vi "FPGA_DIOWritePWMMinHigh.vi"(8 "error in (no error)":errorcluster, 10 "PWMMinHigh":u16=98, 11 "DIODeviceRef In":T1) -> (0 "error out":errorcluster, 3 "DIODeviceRef Out":T1)   [LabVIEW 2017]
uses:
  <vilib>/Rock Robotics/SystemInterfaces/DIO/FPGA_DIODevRef.ctl
  <vilib>/Rock Robotics/SystemInterfaces/System/FPGA_SystemFPGA Ref Global.vi
  <vilib>/Utility/error.llb/Error Cluster From Error Code.vi
  <vilib>/rvi/errors/niLvFpgaAdjustHostInterfaceError.vi
  <vilib>/rvi/interface/nirviReadWriteControl/nirviReadWriteControl.xnode
  <vilib>/Rock Robotics/SystemInterfaces/System/FPGA_SystemFRC FPGA Ref.ctl
  <vilib>/rvi/interface/Simulation/niFpgaSimulationCallBeginRW.vi
  NiFpgaLv.dll
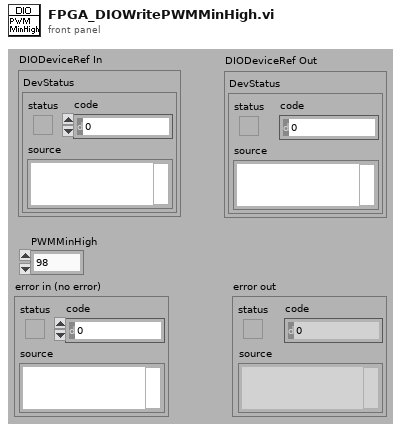
[diagram p1: front panel]
types:
  T1 = typedef "FPGA_DIODevRef.ctl" = cluster{"DevStatus":errorcluster}
  T2 = typedef "FPGA_SystemFRC FPGA Ref.ctl" = refnum<k20>
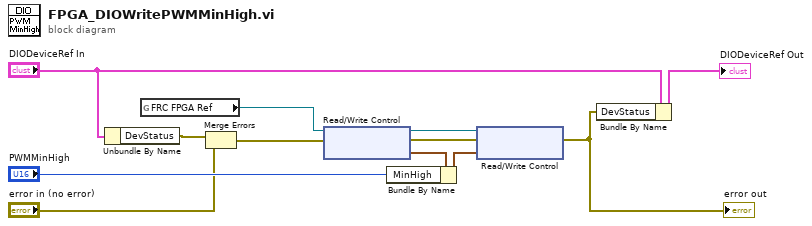
[diagram p0: block diagram]
diagram:
  n1 = Unbundle By Name("DIODeviceRef In") -> ("DevStatus"=w9:errorcluster)
  n2 = global read "FPGA_SystemFPGA Ref Global.vi" "FRC FPGA Ref"() -> (w7:T2)
  n3 = Merge Errors(w9, "error in (no error)") -> (w8:errorcluster)
  n4 = xnode "Read/Write Control"("FPGA VI Reference In"=w7, "error in"=w8) -> ("FPGA VI Reference Out"=w5:T2, "error out"=w6:errorcluster, "PWM.Config"=w4:cluster{"Period":u16, "MinHigh":u16})
  n5 = Bundle By Name(cluster=w4, "MinHigh"="PWMMinHigh") -> (w3:cluster{"Period":u16, "MinHigh":u16})
  n6 = xnode "Read/Write Control"("FPGA VI Reference In"=w5, "error in"=w6, "PWM.Config"=w3) -> ("error out"=w11:errorcluster)  [unwired: 1 out]
  "error out" <- w11
  n7 = Bundle By Name(cluster="DIODeviceRef In", "DevStatus"=w11) -> (→"DIODeviceRef Out":T1)
